vi "SM PRACTICE DFRNT STYLE.vi"() -> ()   [LabVIEW 2020]
panel:
  out "Array":dbl[](array[numeric])
  out "Random Number's":dbl
  in  "stop":bool
  in  "OK Button":bool
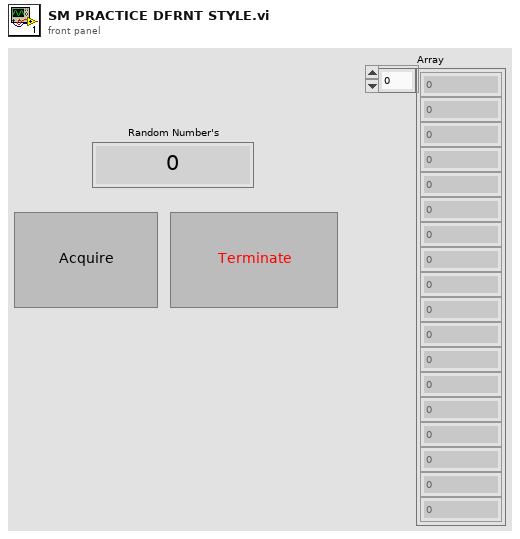
[diagram p1: front panel]
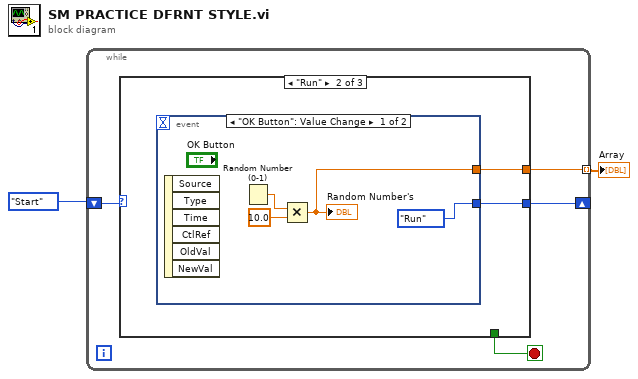
[diagram p0: block diagram]
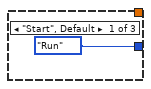
[diagram p2: hidden frame]
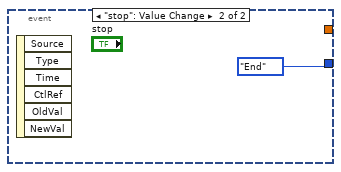
[diagram p3: hidden frame]
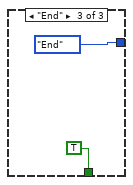
[diagram p4: hidden frame]
diagram:
  n1 = while {
    shift-right: [w5] -> _
    shift-left: enum16{"Start", "Run", "End"}."Start" -> [w6]
    tunnel: [w3] -> w1 mode=indexing
    stop <- w4 stop-if-true
    n2 = case shown="\"Run\"" w6 {
      tunnel: [enum16{"Start", "Run", "End"}."Run" w9 enum16{"Start", "Run", "End"}."End"] -> w5
      tunnel: [_ _ TRUE] -> w4
      tunnel: [_ w8 _] -> w3
      frame "Start", Default {
      }
      frame "Run" {
        n3 = event shown="[0] \"OK Button\": Value Change" {
          selector: _ -> [_ _]
          dyn-events: _ -> [_ _]
          timeout: _ -> [_ _]
          tunnel: [enum16{"Start", "Run", "End"}."Run" enum16{"Start", "Run", "End"}."End"] -> w9
          tunnel: [w10 _] -> w8
          event "OK Button": Value Change {
            n4 = event-data() -> ()  [unwired: 1 in, 6 out]
            n5 = Random Number (0-1)() -> (number: 0 to 1=w13:dbl)
            n6 = Multiply(x=w13, y=10.0) -> (x*y=w10:dbl)
            "Random Number's" <- w10
          }
          event "stop": Value Change {
            n7 = event-data() -> ()  [unwired: 1 in, 6 out]
          }
        }
      }
      frame "End" {
      }
    }
  }
  "Array" <- w1
